vi "Calculate 2D linear spiral.vi"(3 "Start position ax1":dbl format="%.6f", 4 "Start position ax2":dbl format="%.6f", 6 "Range":dbl format="%.2f", 7 "Step size":dbl format="%.2f") -> (10 "Min. pos. ax2":dbl format="%.6f", 11 "Max. pos. ax2":dbl format="%.6f", 12 "1D pos. array ax2":dbl[](array[numeric]) format="%.6f", 14 "1D pos. array ax1":dbl[](array[numeric]) format="%.6f", 15 "Min. pos. ax1":dbl format="%.6f", 16 "Max. pos. ax1":dbl format="%.6f", 17 "No. of steps":i32, 18 "2D intensity array":dbl[][](array[numeric]) format="%.6f")   [LabVIEW 2020]
doc: "Calculates position values for a 2D linear spiral scan and initializes intensity array according to Start position of axes 1 and 2, Step size and Range. The VI returns minimum position, maximum position, No. of steps and initialized 1D position array for axes 1 and 2 and a 2D intensity array."
panel:
  # "Calculates position values for a 2D linear spiral scan and initializes intensity array."
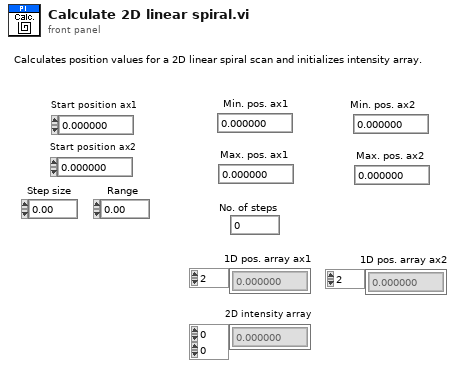
[diagram p1: front panel]
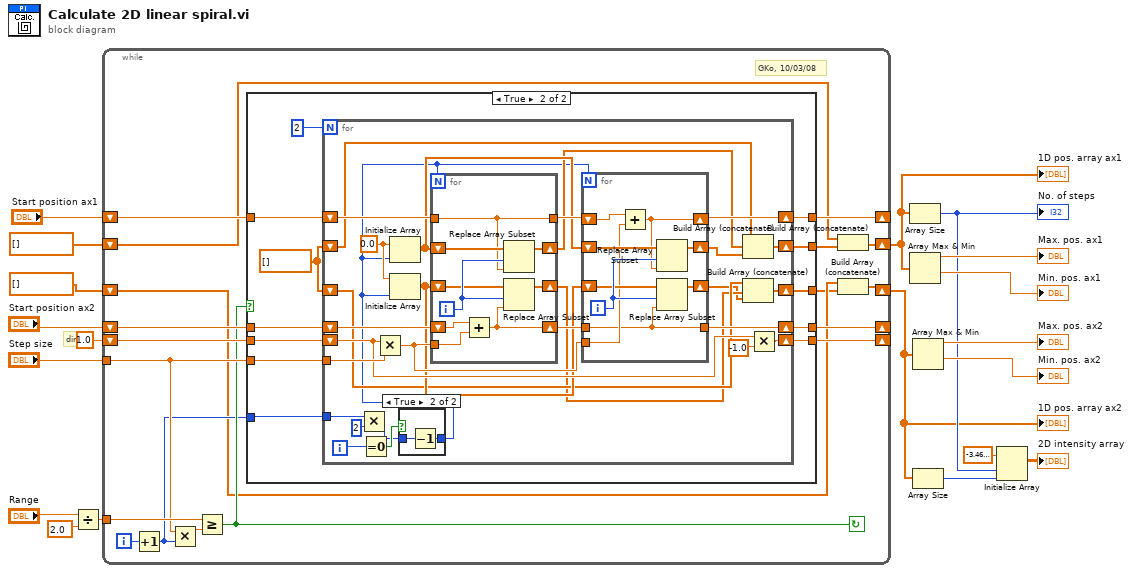
[diagram p0: block diagram]
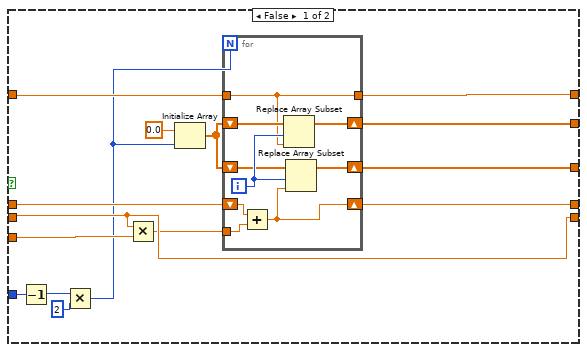
[diagram p2: hidden frame]
diagram:
  # "dir"
  n1 = Divide(x="Range", y=2.0) -> (x/y=w1:dbl)
  n2 = while {
    shift-left: dbl[] [] -> [w25]
    shift-right: [w23] -> w7
    tunnel: "Step size" -> [w32]
    shift-right: [w27] -> _
    shift-left: 1.0 ("y") -> [w31]
    shift-right: [w22] -> w6
    shift-left: dbl[] [] -> [w21]
    shift-right: [w29] -> _
    shift-left: "Start position ax1" -> [w36]
    shift-right: [w28] -> _
    shift-left: "Start position ax2" -> [w35]
    tunnel: w1 -> [w33]
    i -> [w37]
    stop <- w30 continue-if-true
    # "GKo, 10/03/08"
    n3 = Increment(x=w37) -> (x+1=w26:i32)
    n4 = Multiply(x=w32, y=w26) -> (x*y=w34:dbl)
    n5 = Greater Or Equal?(x=w33, y=w34) -> (x >= y?=w30:bool)
    n6 = case shown="True" w30 {
      tunnel: w36 -> [w50 w73]
      tunnel: w35 -> [w47 w72]
      tunnel: w32 -> [w52 w67]
      tunnel: [w49 w71] -> w29
      tunnel: [w46 w70] -> w28
      tunnel: w31 -> [w44 w69]
      tunnel: [w44 w64] -> w27
      tunnel: [w48 w66] -> w24
      tunnel: [w45 w65] -> w20
      tunnel: w26 -> [w51 w62]
      frame False {
        n7 = Decrement(x=w51) -> (x-1=w43:i32)
        n8 = Multiply(x=w43, y=2) -> (x*y=w39:i32)
        n9 = Multiply(x=w44, y=w52) -> (x*y=w38:dbl)
        n10 = Initialize Array(0.0 ("y"), w39) -> (w40:dbl[])
        n11 = for {
          N: w39 -> [_]
          shift-right: [w59] -> w48
          shift-left: w40 -> [w60]
          shift-right: [w57] -> w45
          shift-left: w40 -> [w58]
          tunnel: w50 -> [w54]
          shift-right: [w55] -> w46
          shift-left: w47 -> [w56]
          tunnel: [w54] -> w49
          tunnel: w38 -> [w53]
          i -> [w61]
          n12 = Add(x=w56, y=w53) -> (x+y=w55:dbl)
          n13 = Replace Array Subset(array=w60, new element=w54, index=w61) -> (w59:dbl[])
          n14 = Replace Array Subset(array=w58, new element=w55, index=w61) -> (w57:dbl[])
        }
      }
      frame True {
        w68 = dbl[] []
        n15 = for {
          N: 2 -> [_]
          tunnel: w67 -> [w98]
          shift-right: [w84] -> w66
          shift-left: w68 -> [w87]
          shift-right: [w83] -> w65
          shift-left: w68 -> [w82]
          shift-right: [w92] -> w64
          shift-left: w69 -> [w91]
          shift-right: [w94] -> w71
          shift-left: w73 -> [w100]
          shift-right: [w93] -> w70
          shift-left: w72 -> [w99]
          tunnel: w62 -> [w78]
          i -> [w77]
          w101 = 0.0 ("y")
          n16 = Multiply(x=w78, y=2) -> (x*y=w75:i32)
          n17 = Equal To 0?(x=w77) -> (x = 0?=w76:bool)
          n18 = Multiply(x=w91, y=w98) -> (x*y=w95:dbl)
          n19 = case shown="True" w76 {
            tunnel: w75 -> [w102 w104]
            tunnel: [w102 w103] -> w74
            frame False {
            }
            frame True {
              n20 = Decrement(x=w104) -> (x-1=w103:i32)
            }
          }
          n21 = Initialize Array(w101, w74) -> (w89:dbl[])
          n22 = Initialize Array(w101, w74) -> (w88:dbl[])
          n23 = for {
            N: w74 -> [_]
            shift-right: [w120] -> w86
            shift-left: w89 -> [w121]
            shift-right: [w118] -> w81
            shift-left: w88 -> [w119]
            tunnel: w100 -> [w115]
            shift-right: [w116] -> w97
            shift-left: w99 -> [w117]
            tunnel: [w115] -> w96
            tunnel: w95 -> [w114]
            i -> [w122]
            n24 = Add(x=w117, y=w114) -> (x+y=w116:dbl)
            n25 = Replace Array Subset(array=w121, new element=w115, index=w122) -> (w120:dbl[])
            n26 = Replace Array Subset(array=w119, new element=w116, index=w122) -> (w118:dbl[])
          }
          n27 = for {
            N: w74 -> [_]
            shift-right: [w111] -> w85
            shift-left: w89 -> [w112]
            shift-right: [w109] -> w80
            shift-left: w88 -> [w110]
            shift-right: [w107] -> w94
            shift-left: w96 -> [w108]
            tunnel: w97 -> [w105]
            tunnel: w95 -> [w106]
            tunnel: [w105] -> w93
            i -> [w113]
            n28 = Add(x=w108, y=w106) -> (x+y=w107:dbl)
            n29 = Replace Array Subset(array=w112, new element=w107, index=w113) -> (w111:dbl[])
            n30 = Replace Array Subset(array=w110, new element=w105, index=w113) -> (w109:dbl[])
          }
          n31 = Build Array (concatenate)(w87, w86, w85) -> (w84:dbl[])
          n32 = Build Array (concatenate)(w82, w81, w80) -> (w83:dbl[])
          n33 = Multiply(x=w91, y=-1.0) -> (x*y=w92:dbl)
        }
      }
    }
    n34 = Build Array (concatenate)(w25, w24) -> (w23:dbl[])
    n35 = Build Array (concatenate)(w21, w20) -> (w22:dbl[])
  }
  "1D pos. array ax1" <- w7
  "1D pos. array ax2" <- w6
  n36 = Array Size(array=w7) -> (size(s)=w9:i32)
  "No. of steps" <- w9
  n37 = Array Max & Min(array=w7) -> (max value=→"Max. pos. ax1":dbl, min value=→"Min. pos. ax1":dbl)  [unwired: 2 out]
  n38 = Array Max & Min(array=w6) -> (max value=→"Max. pos. ax2":dbl, min value=→"Min. pos. ax2":dbl)  [unwired: 2 out]
  n39 = Array Size(array=w6) -> (size(s)=w8:i32)
  n40 = Initialize Array(-3.469446951953614e-18 ("Element Data"), w9, w8) -> (→"2D intensity array":dbl[][])
